vi "My_Method_Password_Lock.vi"() -> ()   [LabVIEW 2026]
panel:
  in  "Keypad":T1
  out "Imagine it is a Buzzer":bool
  out "?":string
  out "7-segment":T2
  out "Opened":bool
  in  "stop 2":bool
  # "D submits \nC clears if a typo occured - as an extra\nThe password is 5681"
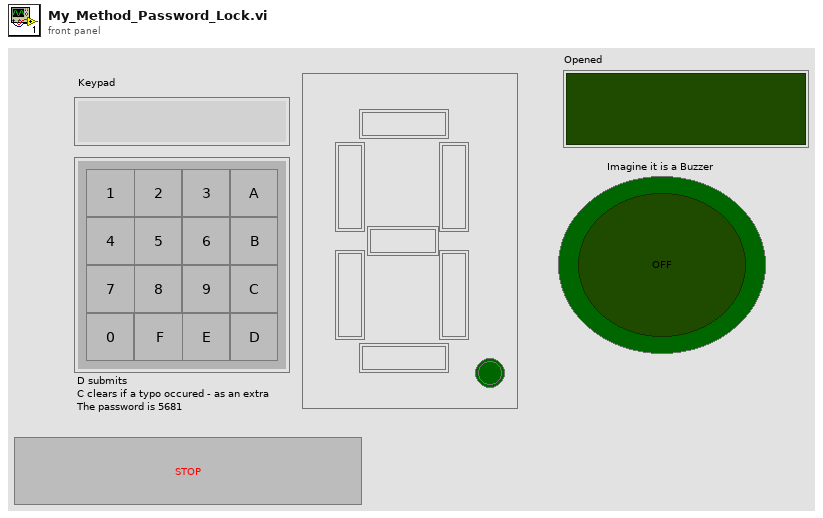
[diagram p1: front panel]
types:
  T1 = cluster{"0":bool, "1":bool, "2":bool, "3":bool, "4":bool, "5":bool, "6":bool, "7":bool, "8":bool, "9":bool, "F":bool, "E":bool, "A":bool, "B":bool, "C":bool, "D":bool}
  T2 = cluster{"a":bool, "b":bool, "c":bool, "d":bool, "e":bool, "f":bool, "g":bool, "DP":bool}
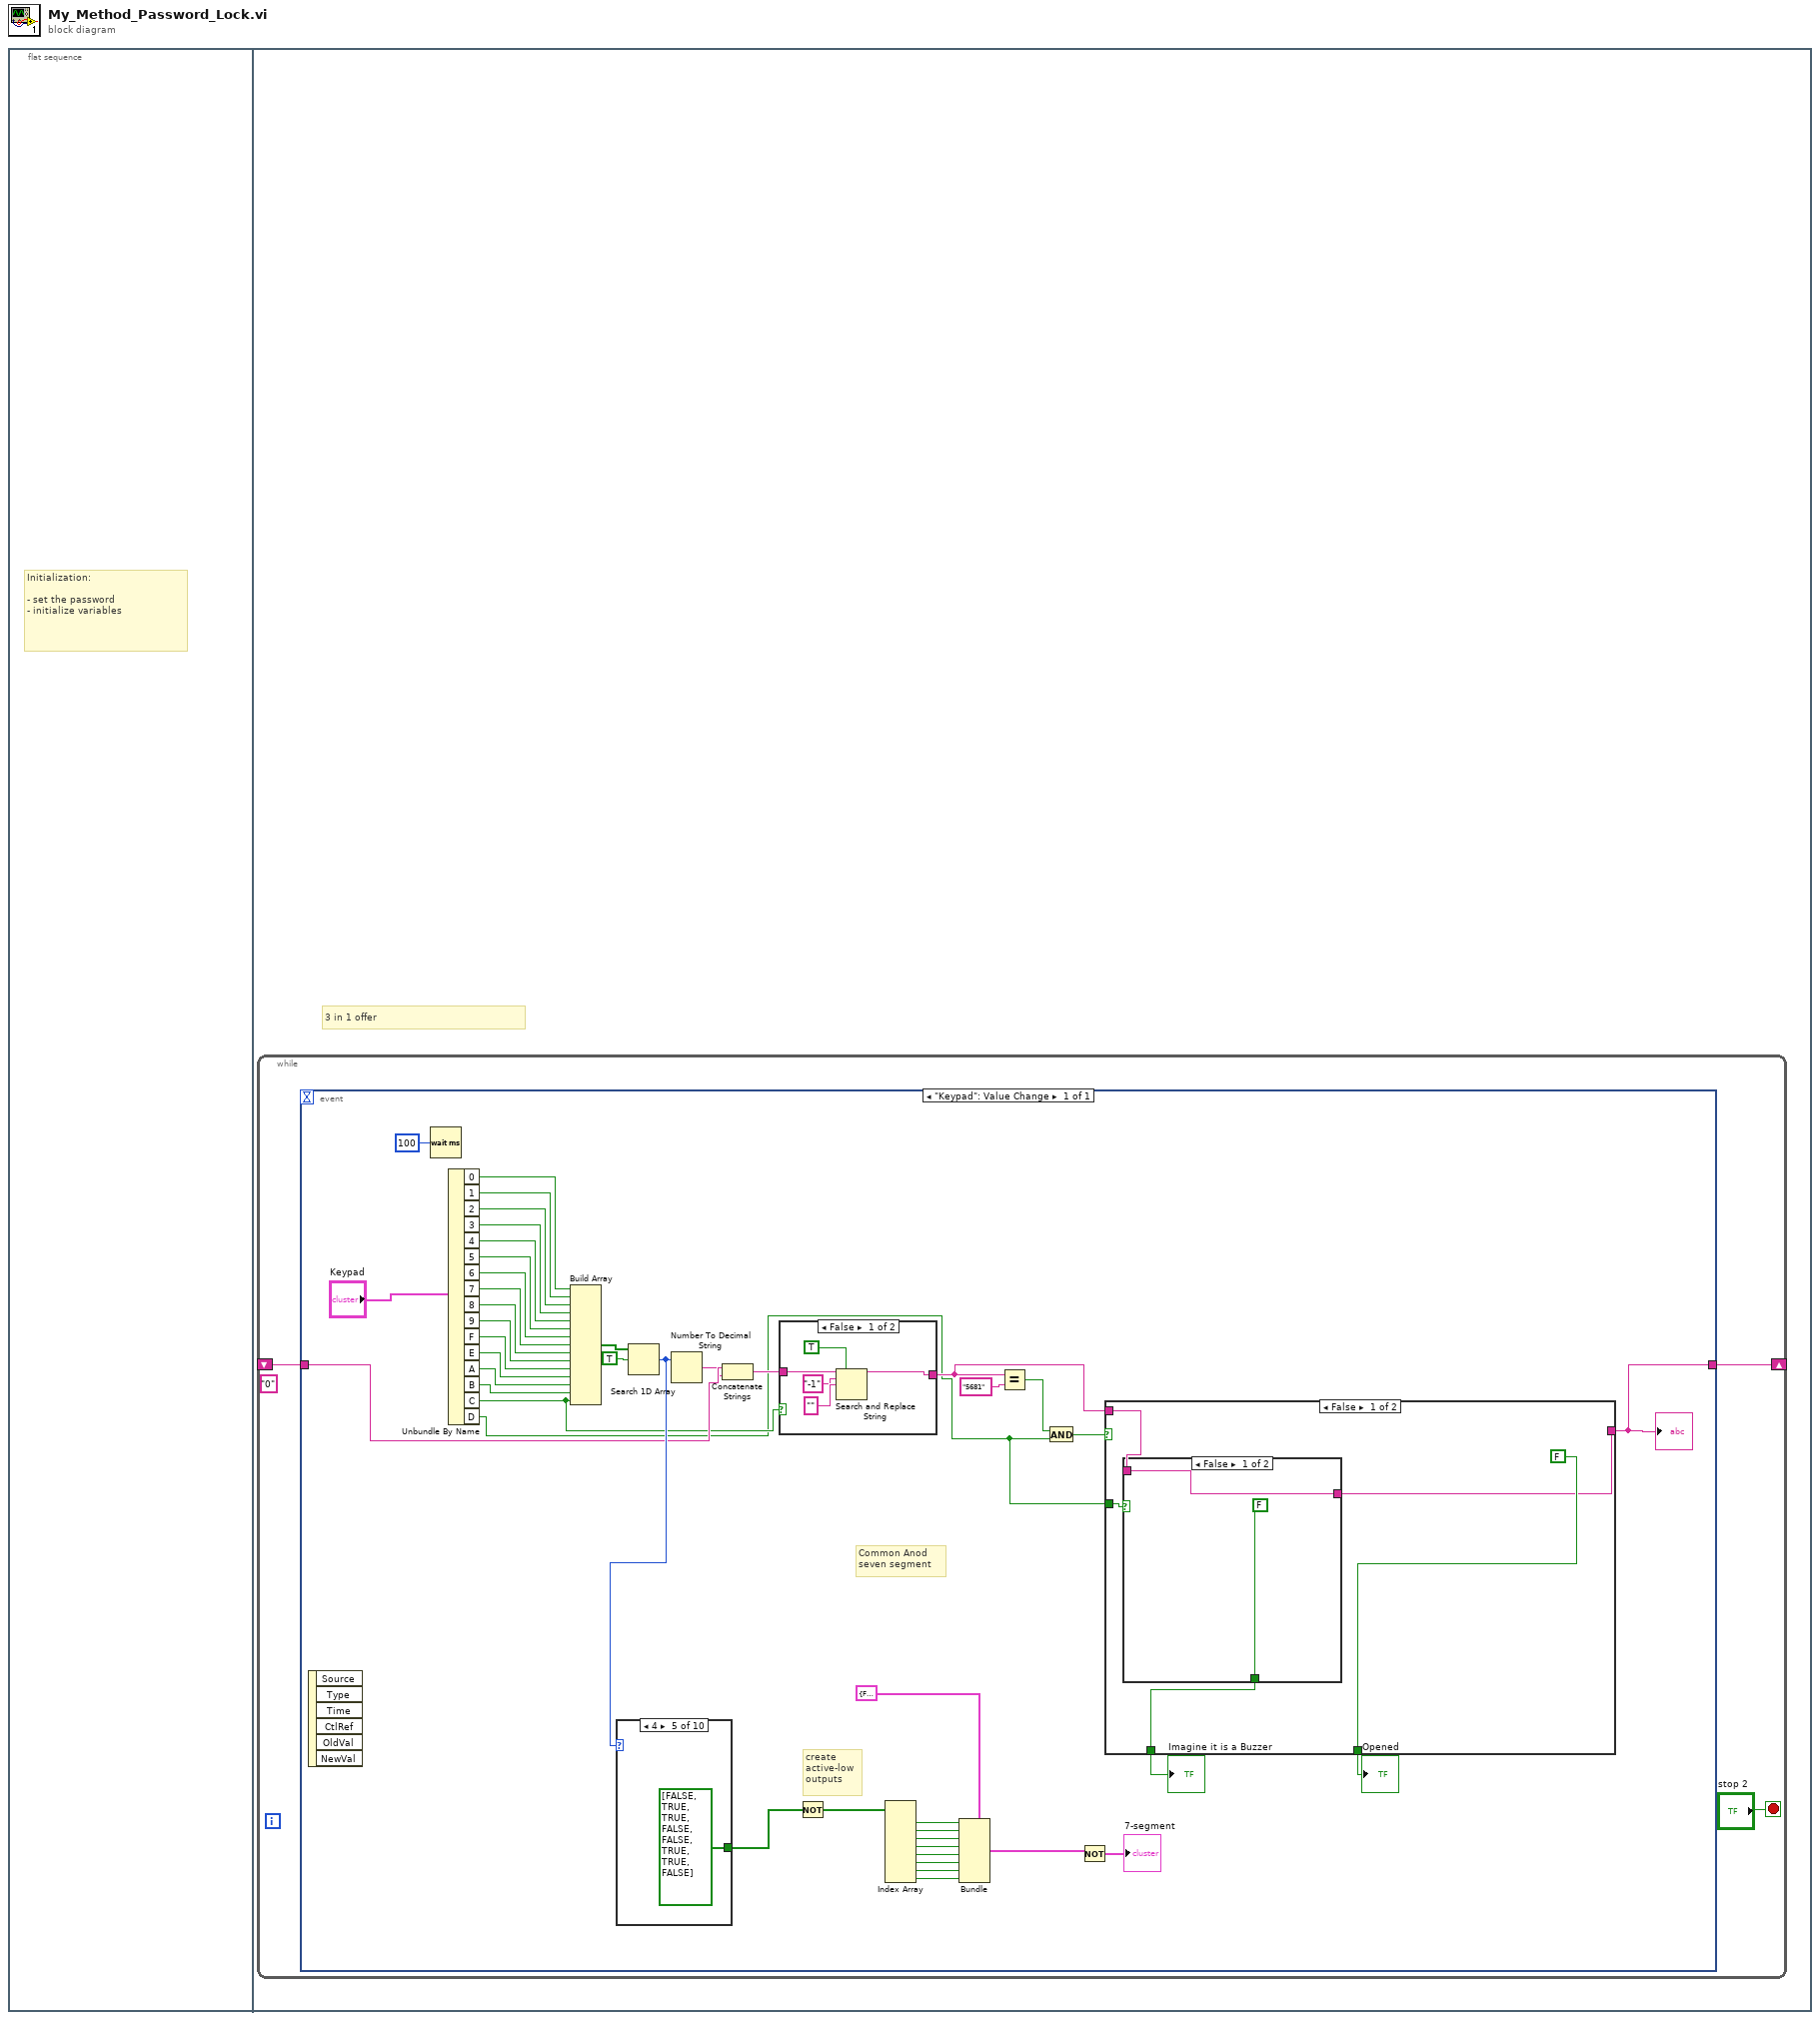
[diagram p0: block diagram]
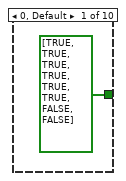
[diagram p2: hidden frame]
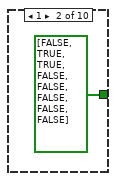
[diagram p3: hidden frame]
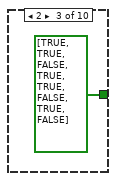
[diagram p4: hidden frame]
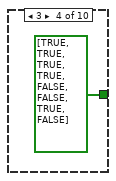
[diagram p5: hidden frame]
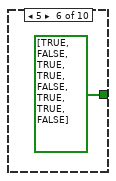
[diagram p6: hidden frame]
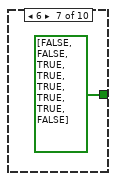
[diagram p7: hidden frame]
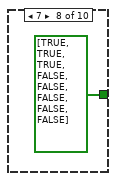
[diagram p8: hidden frame]
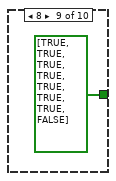
[diagram p9: hidden frame]
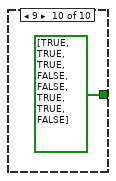
[diagram p10: hidden frame]
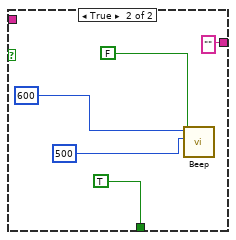
[diagram p11: hidden frame]
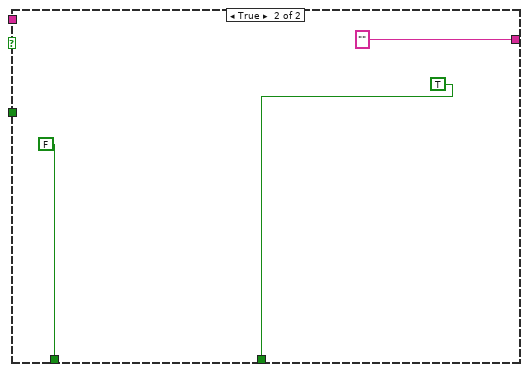
[diagram p12: hidden frame]
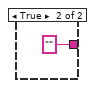
[diagram p13: hidden frame]
diagram:
  n1 = flat-sequence {
    frame #0 {
      # "Initialization:\n\n- set the password\n- initialize variables"
    }
    frame #1 {
      # "3 in 1 offer"
      n2 = while {
        shift-right: [w2] -> _
        shift-left: _ -> [w1]
        stop <- "stop 2" stop-if-true
        (unwired) "0"
        n3 = event shown="[0] \"Keypad\": Value Change" {
          selector: _ -> [_]
          dyn-events: _ -> [_]
          timeout: _ -> [_]
          tunnel: [w7] -> w2
          tunnel: w1 -> [w11]
          event "Keypad": Value Change {
            # "Common Anod \nseven segment"
            # "create\nactive-low\noutputs"
            n4 = event-data() -> ()  [unwired: 1 in, 6 out]
            n5 = Wait (ms)(milliseconds to wait=u32 100) -> ()  [unwired: 1 out]
            n6 = Unbundle By Name("Keypad") -> ("0"=w29:bool, "1"=w28:bool, "2"=w27:bool, "3"=w26:bool, "4"=w25:bool, "5"=w24:bool, "6"=w23:bool, "7"=w22:bool, "8"=w21:bool, "9"=w20:bool, "F"=w19:bool, "E"=w18:bool, "A"=w17:bool, "B"=w16:bool, "C"=w8:bool, "D"=w6:bool)
            n7 = Build Array(w29, w28, w27, w26, w25, w24, w23, w22, w21, w20, w19, w18, w17, w16, w8) -> (w15:bool[])
            n8 = Search 1D Array(1D array=w15, element=TRUE) -> (index of element=w14:i32)  [unwired: 1 in]
            n9 = case shown="4" w14 {
              tunnel: [bool[] [TRUE, TRUE, TRUE, TRUE, TRUE, TRUE, FALSE, FALSE] ("LED segments 2") bool[] [FALSE, TRUE, TRUE, FALSE, FALSE, FALSE, FALSE, FALSE] ("LED segments 2") bool[] [TRUE, TRUE, FALSE, TRUE, TRUE, FALSE, TRUE, FALSE] ("LED segments 2") bool[] [TRUE, TRUE, TRUE, TRUE, FALSE, FALSE, TRUE, FALSE] ("LED segments 2") bool[] [FALSE, TRUE, TRUE, FALSE, FALSE, TRUE, TRUE, FALSE] ("LED segments 2") bool[] [TRUE, FALSE, TRUE, TRUE, FALSE, TRUE, TRUE, FALSE] ("LED segments 2") bool[] [FALSE, FALSE, TRUE, TRUE, TRUE, TRUE, TRUE, FALSE] ("LED segments 2") bool[] [TRUE, TRUE, TRUE, FALSE, FALSE, FALSE, FALSE, FALSE] ("LED segments 2") bool[] [TRUE, TRUE, TRUE, TRUE, TRUE, TRUE, TRUE, FALSE] ("LED segments 2") bool[] [TRUE, TRUE, TRUE, FALSE, FALSE, TRUE, TRUE, FALSE] ("LED segments 2")] -> w41
              frame 0, Default {
              }
              frame 1 {
              }
              frame 2 {
              }
              frame 3 {
              }
              frame 4 {
              }
              frame 5 {
              }
              frame 6 {
              }
              frame 7 {
              }
              frame 8 {
              }
              frame 9 {
              }
            }
            n10 = Number To Decimal String(number=w14) -> (decimal integer string=w10:string)  [unwired: 1 in]
            n11 = Concatenate Strings(w11, w10) -> (w13:string)
            n12 = case shown="False" w8 {
              tunnel: w13 -> [w75 _]
              tunnel: [w73 ""] -> w12
              frame False {
                n13 = Search and Replace String(replace all?=TRUE ("element"), input string=w75, search string="-1", replace string="") -> (result string=w73:string)  [unwired: 4 in, 3 out]
              }
              frame True {
              }
            }
            n14 = Not(x=w41) -> (.not. x?=w42:bool[])
            n15 = Index Array "Index Array"(array=w42) -> (element #1=w40:bool, element #2=w39:bool, element #3=w38:bool, element #4=w37:bool, element #5=w36:bool, element #6=w35:bool, element #7=w34:bool, element #8=w33:bool)  [unwired: 8 in]
            n16 = Bundle(cluster=T2 {"a"=FALSE, "b"=FALSE, "c"=FALSE, "d"=FALSE, "e"=FALSE, "f"=FALSE, "g"=FALSE, "DP"=FALSE} ("7-segment"), "a"=w40, "b"=w39, "c"=w38, "d"=w37, "e"=w36, "f"=w35, "g"=w34, "DP"=w33) -> (w31:T2)
            n17 = Equal?(x=w12, y="5681") -> (x = y?=w44:bool)
            n18 = And(x=w44, y=w6) -> (x .and. y?=w43:bool)
            n19 = Not(x=w31) -> (.not. x?=→"7-segment":T2)
            n20 = case shown="False" w43 {
              tunnel: w12 -> [w59 _]
              tunnel: [w60 FALSE] -> w4
              tunnel: [FALSE TRUE] -> w9
              tunnel: [w58 ""] -> w7
              tunnel: w6 -> [w61 _]
              frame False {
                n21 = case shown="False" w61 {
                  tunnel: [FALSE TRUE] -> w60
                  tunnel: w59 -> [w63 _]
                  tunnel: [w63 ""] -> w58
                  frame False {
                  }
                  frame True {
                    n22 = call <vilib>:"Beep.vi"("use system alert? (T)"=FALSE, "duration (msec)"=500, "frequency (Hz)"=600) -> ()  [unwired: 9 in]
                  }
                }
              }
              frame True {
              }
            }
            "Imagine it is a Buzzer" <- w4
            "Opened" <- w9
            "?" <- w7
          }
        }
      }
    }
  }
